vi "take_snapshots.vi"() -> ()   [LabVIEW 2019]
uses:
  <vilib>/userDefined/High Color/IMAQdx.ctl
  <vilib>/vision/driver/IMAQdx.llb/IMAQdx Attribute Type.ctl
  <vilib>/vision/Management.llb/Cast Image 2 Method.ctl
  <vilib>/DAQmx/write.llb/DAQmx Write (Analog DBL 1Chan 1Samp).vi
  <vilib>/DAQmx/read.llb/DAQmx Read (Analog DBL 1Chan 1Samp).vi
  <vilib>/Analysis/baseanly.llb/Mean (DBL).vi
  <vilib>/DAQmx/create/channels.llb/DAQmx Create Channel (AO-Voltage-Basic).vi
  <vilib>/DAQmx/miscellaneous.llb/DAQmx Fill In Error Info.vi
  <vilib>/DAQmx/create/channels.llb/DAQmx Create Channel (AI-Temperature-Thermocouple).vi
  <vilib>/vision/driver/NI_Vision_Acquisition_Software.lvlib
  <resource>/objmgr/imaqdx.rc
  <vilib>/vision/NI_Vision_Development_Module.lvlib
  <vilib>/Analysis/NI_AALBase.lvlib
panel:
  in  "file path (PID voltage)":path
  in  "PID Control 2":bool
  in  "Desired \nTemperature":dbl=20.0 format="%#_13g"
  in  "DC power supply":refnum<visa-resource-name>="COM3"
  out "voltage monitoring constant":dbl format="%#.2g"
  in  "exit PID loop":bool
  in  "Experiment duration\n(min)":dbl
  in  "Snapshot Period\n (min per snapshot)":dbl
  out "Video":bool
  in  "Action":i32(listbox)=1
  out "meanIntensity":dbl[](array[numeric])
  out "varLaplacian":dbl[](array[numeric])
  out "mean":dbl
  out "variance":dbl
  out "Avg Intensity":dbl(graph)=4.716017316017316
  in  "Activate":bool
  out "Var of Laplacian":dbl(graph)=63.940469067936796
  in  "ROI":T1={"Global Rectangle"=[], "Contours"=[{"Contour Type"=0, "ROI Type"=3, "Points"=[231, 86, 235, 90]}, {"Contour Type"=0, "ROI Type"=3, "Points"=[193, 50, 270, 125]}]}
  in  "error in":errorcluster
  in  "File path for video":string="C:\\Users\\Aniket\\Desktop\\mCherry_calibration\\new_lens\\laser_calibration\\laser_and_heating\\"
  in  "Laser profile file path":path=path "C:/Users/Aniket/Desktop/mCherry_calibration/new_lens/laser_calibration/laser_profiles/new_profile.txt"
  in  "Trigger Laser":bool
  in  "Image file path \n(Do not add specify file extension - set to png)":path=path "C:/Users/Aniket/Desktop/mCherry_calibration/new_lens/laser_calibration/laser_profiles.txt"
  out "Current \nTemperature":dbl format="%0.2f"
  out "?":dbl[](graph)=[37.63236695538445]
  out "error out 7":errorcluster
  out "error out 6":errorcluster
  out "error out 5":errorcluster
  out "Exposure Time":dbl
  in  "ON/OFF":bool
  out "error out 3":errorcluster
  in  "LED":dbl(slide) scale=0.0..10.0
  in  "Refresh":bool
  out "Record":bool
  out "Processed Frames per Second":dbl
  out "Acquired Frame Rate":dbl
  out "error out":errorcluster
  out "Camera Display":T2(plugin-control) caption="Image Out"
  in  "Frame Rate":dbl=20.0
  out "Attribute Information Array":T4(array[cluster])
  in  "Session In":T5="cam0"
  # "Camera frame"
  # "Observer frame"
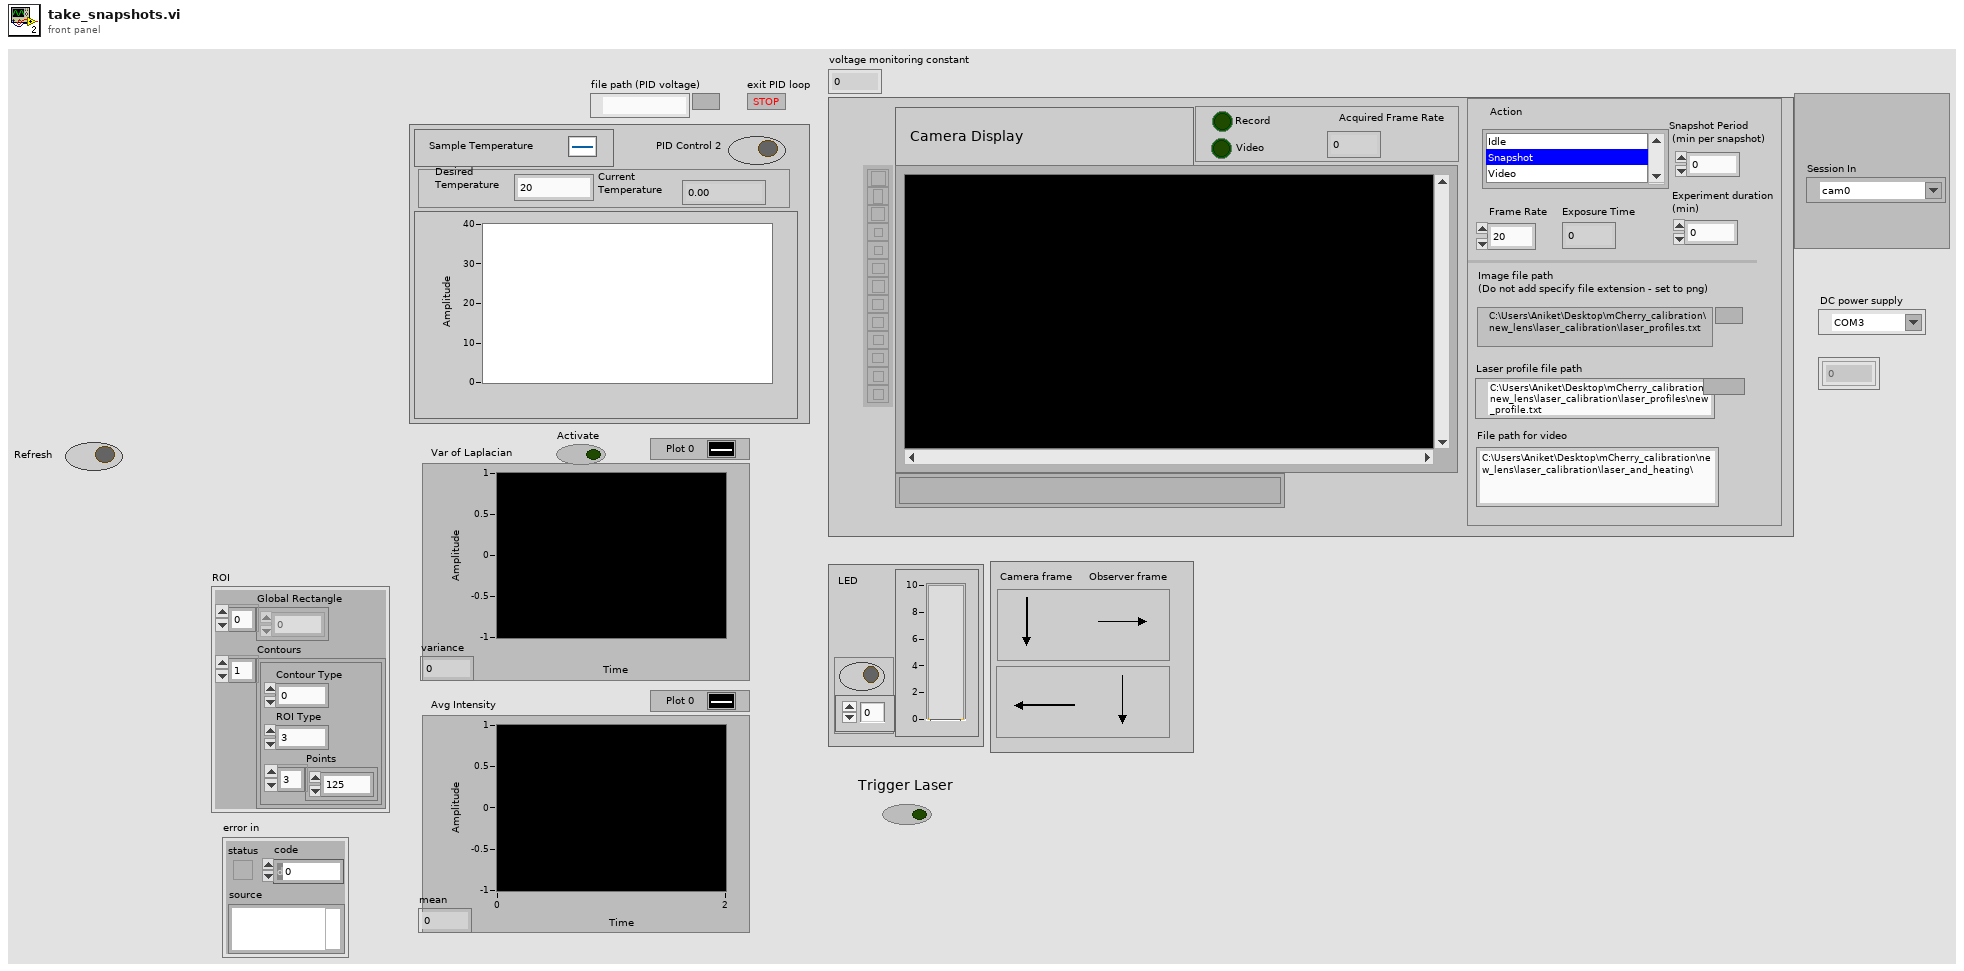
[diagram p1: front panel]
types:
  T1 = cluster{"Global Rectangle":i32[], "Contours":cluster{"Contour Type":u32, "ROI Type":u32, "Points":i32[]}[]}
  T2 = typedef "IMAQ Image.ctl" = refnum<image>
  T3 = typedef "NI_Vision_Acquisition_Software.lvlib/IMAQdx Attribute Type.ctl" = enum32{"U32", "I64", "DBL", "String", "Enum", "Bool", "Command"}
  T4 = cluster{"Attribute Type":T3, "Readable":bool, "Writable":bool, "Attribute Name":string}[]
  T5 = typedef "IMAQdx.ctl" = refnum<k21>
  T6 = enum16{"open", "replace", "create", "open or create", "replace or create", "replace or create with confirmation"}
  T7 = typedef "Image Type" = u32
  T8 = typedef "ROI Descriptor" = cluster{"Global Rectangle":i32[], "Contours":cluster{"ID":enum32{"External", "Internal"}, "Type":u32, "Coordinates":i32[]}[]}
  T9 = typedef "IMAQ Rectangle" = cluster{"Left":i32, "Top":i32, "Right":i32, "Bottom":i32, "Rotation":dbl}
  T10 = typedef "Cast Image 2 Method.ctl" = u32
  T11 = typedef "IMAQ AVI2 Refnum.ctl" = refnum<k20>
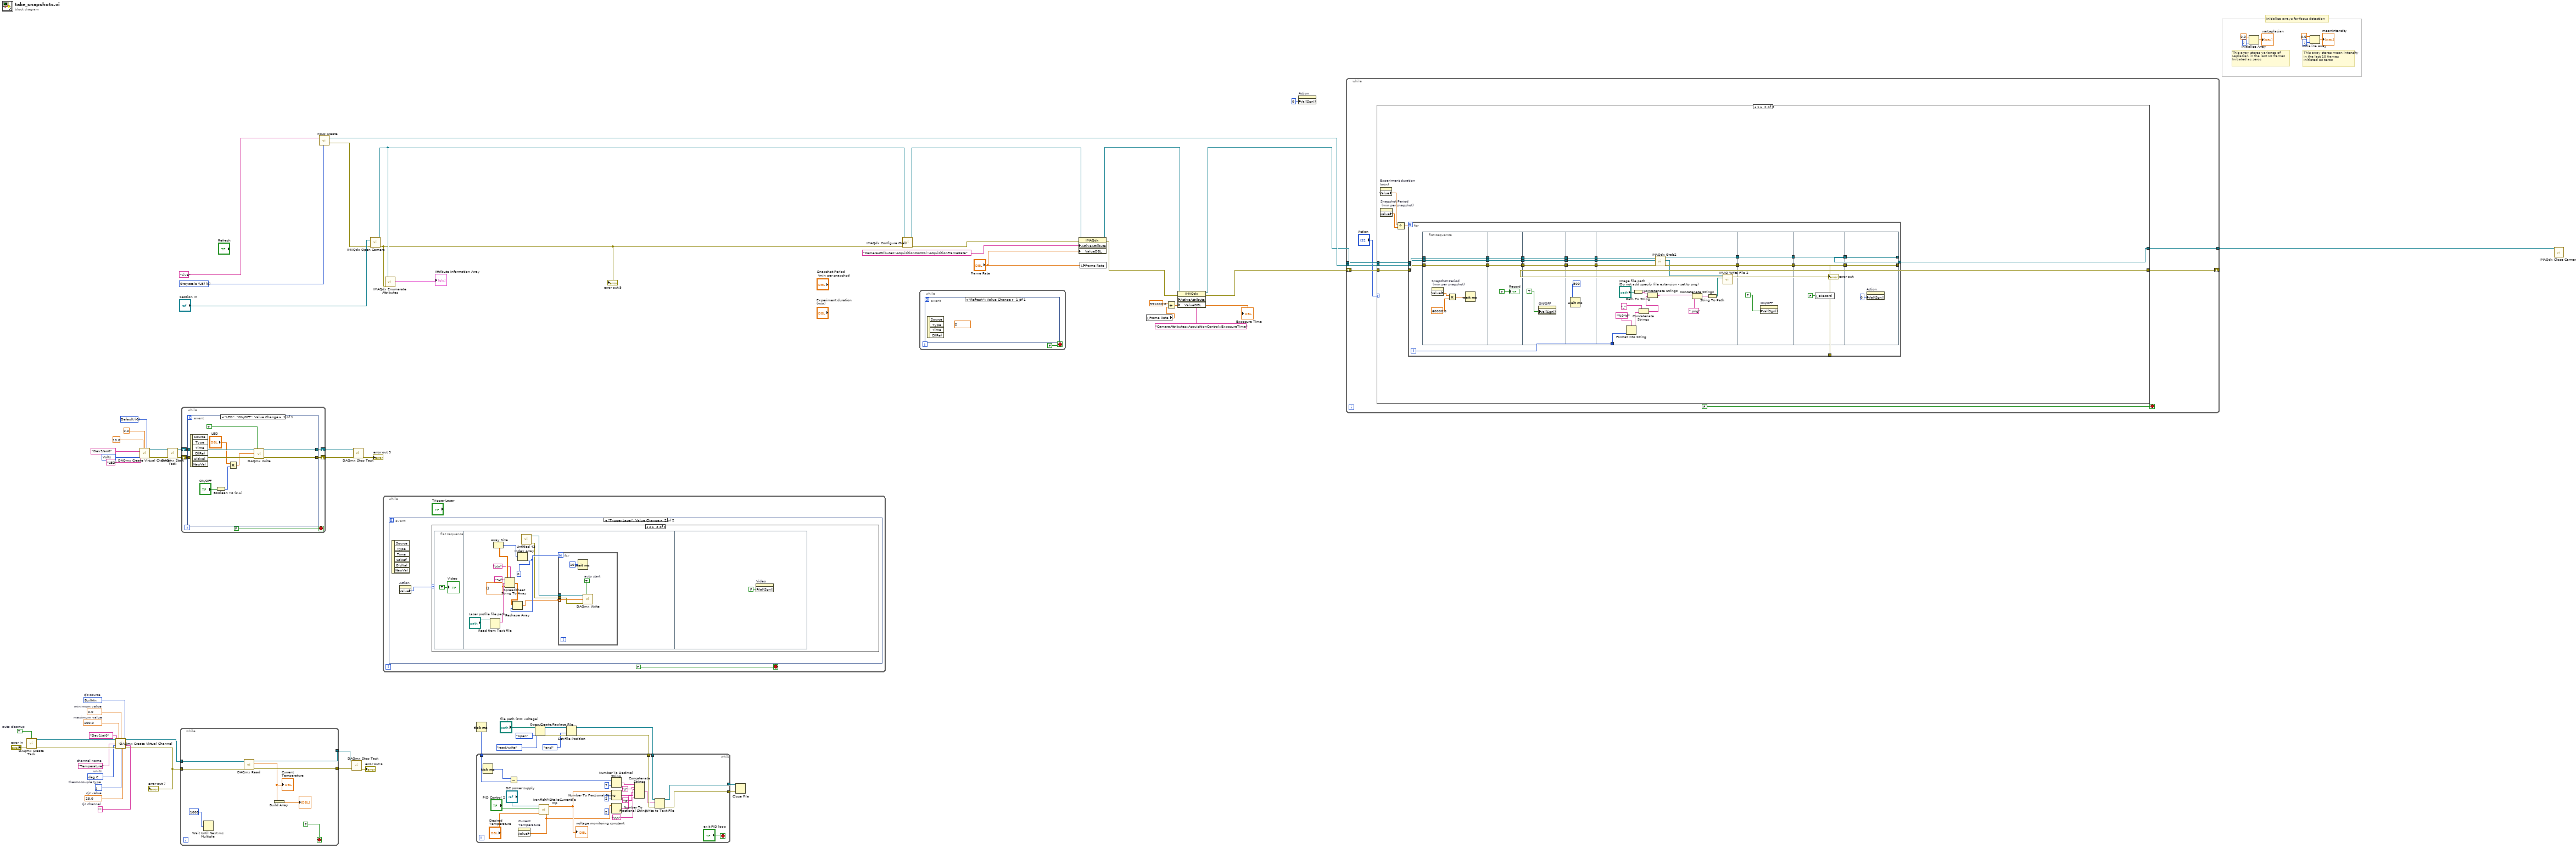
[diagram p0: block diagram]
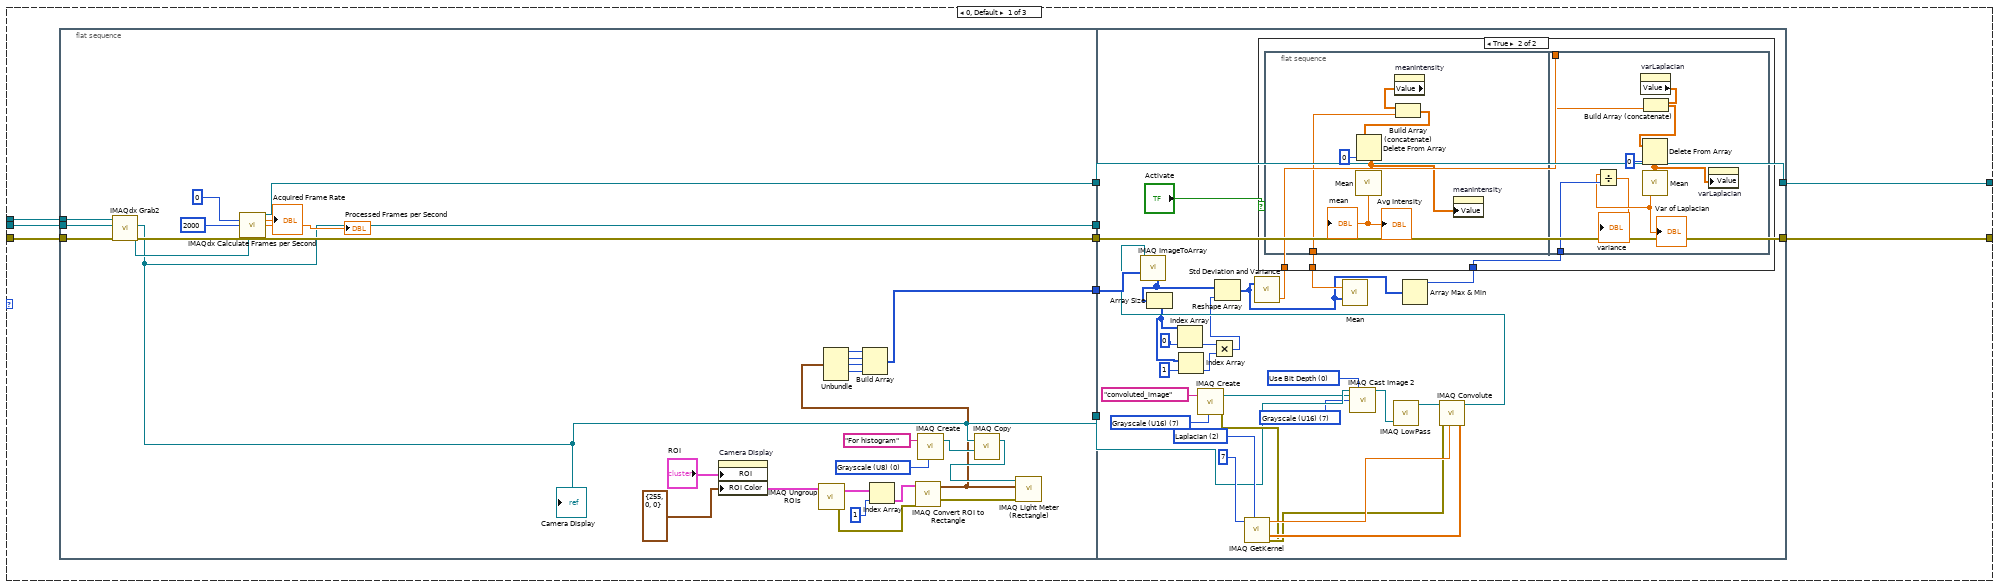
[diagram p2: hidden frame]
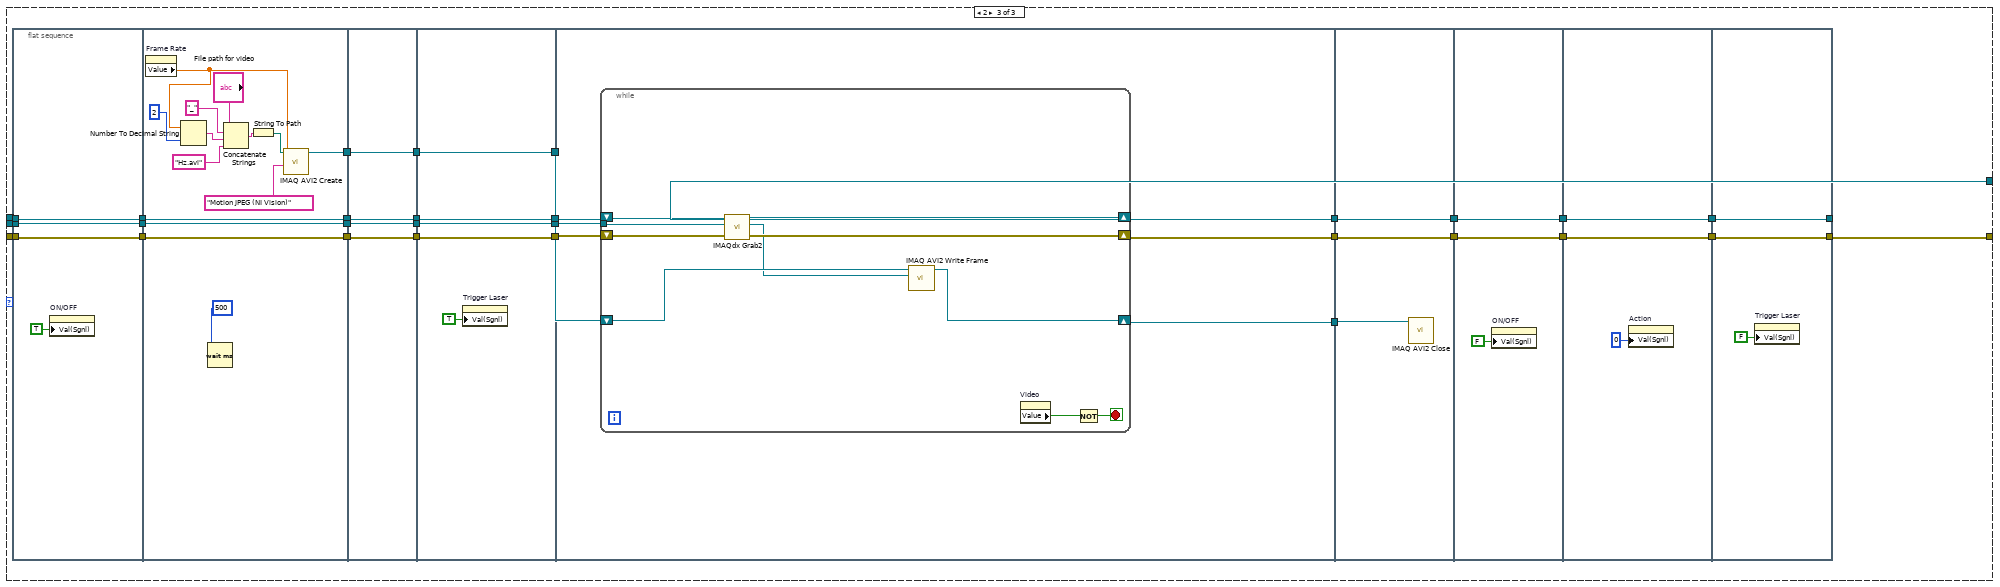
[diagram p4: hidden frame]
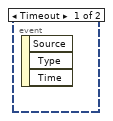
[diagram p5: hidden frame]
diagram:
  w24 = 10200 items=["Built-In"=10200, "Constant Value"=10116, "Channel"=10113]  # cjc source
  w26 = ""  # cjc channel
  w27 = 25.0  # cjc value
  w28 = 10072 items=["J"=10072, "K"=10073, "N"=10077, "R"=10082, "S"=10085, "T"=10086, "B"=10047, "E"=10055]  # thermocouple type
  w29 = 10143 items=["deg C"=10143, "deg F"=10144, "Kelvins"=10325, "deg R"=10145, "From Custom Scale"=10065]  # units
  w25 = "Temperature"  # channel name
  w30 = 0.0  # minimum value
  w31 = 100.0  # maximum value
  w33 = TRUE  # auto cleanup
  w56 = 10348 items=["Volts"=10348, "From Custom Scale"=10065] ("units")
  w58 = -1 items=["Default"=-1, "RSE"=10083, "NRSE"=10078, "Differential"=10106, "Pseudodifferential"=12529] ("input terminal configuration")
  w69 = T7 0 items=["Grayscale (U8)", "Grayscale (I16)", "Grayscale (SGL)", "Complex (CSG)", "RGB (U32)", "HSL (U32)", "RGB (U64)", "Grayscale (U16)"] ("Image Type")
  # "Initialize arrays for focus detection"
  # "This array stores mean intensity in the last 10 frames\nInitiated as zeros"
  # "This array stores variance of Laplacian in the last 10 frames\nInitiated as zeros"
  n1 = call <vilib>:"DAQmx Create Task.vi"("auto cleanup"=w33, "error in"="error in") -> ("task out"=w32:refnum<k21>, "error out"=w34:errorcluster)  [unwired: 12 in]
  n2 = call-poly <vilib>:"DAQmx Create Virtual Channel.vi"("task in"=w32, "maximum value"=w31, "minimum value"=w30, "physical channels"=tag "Dev1/ai0", "cjc source"=w24, "name to assign"=w25, "units"=w29, "cjc channel"=w26, "error in"=w34, "thermocouple type"=w28, "cjc value"=w27) -> ("task out"=w23:refnum<k21>, "error out"=w22:errorcluster)  [unwired: 3 in]
  "error out 7" <- w22
  n3 = call-poly <vilib>:"DAQmx Create Virtual Channel.vi"("maximum value"=10.0, "minimum value"=0.0, "output terminal configuration"=w58, "physical channels"=tag "Dev3/ao0", "name to assign"="LED", "units"=w56) -> ("task out"=w54:refnum<k21>, "error out"=w53:errorcluster)  [unwired: 8 in]
  n4 = call <vilib>:"DAQmx Start Task.vi"("task/channels in"=w54, "error in"=w53) -> ("task out"=w52:refnum<k21>, "error out"=w51:errorcluster)  [unwired: 12 in]
  n5 = while {
    tunnel: w23 -> [w78]
    tunnel: w22 -> [w77]
    tunnel: [w76] -> w38
    tunnel: [w75] -> w37
    stop <- FALSE ("Monitor Temperature") stop-if-true
    n6 = Wait Until Next ms Multiple(millisecond multiple=u32 1000 ("millisecond timer value")) -> ()  [unwired: 1 out]
    n7 = call-poly <vilib>:"DAQmx Read.vi"("task/channels in"=w78, "error in"=w77) -> ("task out"=w76:refnum<k21>, "data"=w72:dbl, "error out"=w75:errorcluster)  [unwired: 11 in]
    "Current \nTemperature" <- w72
    n8 = Build Array(w72) -> (→"?":dbl[])
  }
  n9 = while {
    shift-right: [w82] -> w50
    shift-left: w52 -> [w84]
    shift-right: [w81] -> w49
    shift-left: w51 -> [w83]
    stop <- FALSE stop-if-true
    n10 = event shown="[0] \"LED\", \"ON/OFF\": Value Change" {
      selector: _ -> [_]
      dyn-events: _ -> [_]
      timeout: _ -> [_]
      tunnel: w84 -> [w93]
      tunnel: w83 -> [w92]
      tunnel: [w91] -> w82
      tunnel: [w90] -> w81
      event "LED", "ON/OFF": Value Change {
        n11 = event-data() -> ()  [unwired: 1 in, 6 out]
        n12 = Boolean To (0,1)(Boolean="ON/OFF") -> (0, 1=w86:i16)
        n13 = Multiply(x="LED", y=w86) -> (x*y=w85:dbl)
        n14 = call-poly <vilib>:"DAQmx Write.vi"("task/channels in"=w93, "auto start"=TRUE, "data"=w85, "error in"=w92) -> ("task out"=w91:refnum<k21>, "error out"=w90:errorcluster)  [unwired: 9 in, 1 out]
      }
    }
  }
  n15 = call "IMAQ Create"("Image Name"="Live", "Image Type"=w69) -> ("New Image"=w63:T2, "error out"=w62:errorcluster)  [unwired: 3 in]
  n16 = call <vilib>:"DAQmx Stop Task.vi"("task/channels in"=w38, "error in"=w37) -> ("error out"=→"error out 6":errorcluster)  [unwired: 12 in, 1 out]
  n17 = call <vilib>:"DAQmx Stop Task.vi"("task/channels in"=w50, "error in"=w49) -> ("error out"=→"error out 3":errorcluster)  [unwired: 12 in, 1 out]
  n18 = call <vilib>:"IMAQdx Open Camera.vi"("error in"=w62, "Session In"="Session In") -> ("error out"=w67:errorcluster, "Session Out"=w68:T5)  [unwired: 8 in]
  "error out 5" <- w67
  n19 = while {
    stop <- FALSE stop-if-true
    n20 = event shown="[1] \"Trigger Laser\": Value Change" {
      selector: _ -> [_ _]
      dyn-events: _ -> [_ _]
      timeout: _ -> [_ _]
      event Timeout {
        n21 = event-data() -> ()  [unwired: 1 in, 3 out]
      }
      event "Trigger Laser": Value Change {
        n22 = event-data() -> ()  [unwired: 1 in, 6 out]
        n23 = property on="Action" class="LstBox (strict)"() -> ("Value"=w95:i32)  [unwired: 2 in, 2 out]
        n24 = case shown="2" w95 {
          frame 0, Default {
          }
          frame 1 {
          }
          frame 2 {
            n25 = flat-sequence {
              frame #0 {
                "Video" <- TRUE ("Video")
              }
              frame #1 {
                n26 = Read from Text File(file (use dialog)="Laser profile file path") -> (text=w104:string)  [unwired: 3 in, 3 out]
                n27 = Spreadsheet String To Array(delimiter (Tab)="\r\n", format string="%f", spreadsheet string=w104, array type (2D Dbl)=dbl[][] []) -> (array=w106:dbl[][])
                n28 = Array Size(array=w106) -> (size(s)=w105:i32[])
                n29 = Index Array(array=w105, index=0) -> (element=w108:i32)
                n30 = Reshape Array(w106, w108) -> (w107:dbl[])
                n31 = call "Untitled 43.vi"() -> ("error out"=w97:errorcluster, "task out"=w98:refnum<k21>)  [unwired: 10 in]
                n32 = for {
                  N: w108 -> [_]
                  tunnel: w107 -> [w109] mode=indexing
                  tunnel: w98 -> [w111]
                  tunnel: w97 -> [w110]
                  w112 = TRUE  # auto start
                  n33 = Wait (ms)(milliseconds to wait=u32 10) -> ()  [unwired: 1 out]
                  n34 = call-poly <vilib>:"DAQmx Write.vi"("task/channels in"=w111, "auto start"=w112, "data"=w109, "error in"=w110) -> ()  [unwired: 9 in, 3 out]
                }
              }
              frame #2 {
                n35 = property on="Video" class="Bool (strict)"("Val(Sgnl)"=FALSE ("Value (Signaling)")) -> ()  [unwired: 2 in, 2 out]
              }
            }
          }
        }
      }
    }
  }
  n36 = call <vilib>:"IMAQdx Enumerate Attributes.vi"("error in"=w67, "Session In"=w68) -> ("Attribute Information Array"=→"Attribute Information Array":T4)  [unwired: 7 in, 2 out]
  n37 = Tick Count (ms)() -> (millisecond timer value=w11:u32)
  n38 = Open/Create/Replace File(file path (use dialog)="file path (PID voltage)", operation (0:open)=T6."open", access (0:read/write)=enum16{"read/write", "read-only", "write-only"}."read/write") -> (refnum out=w7:refnum<file>, error out=w8:errorcluster)  [unwired: 3 in, 1 out]
  n39 = Set File Position(refnum=w7, from (0:start)=enum16{"start", "end", "current"}."end", error in=w8) -> (refnum out=w5:refnum<file>, error out=w4:errorcluster)  [unwired: 1 in]
  n40 = while {
    tunnel: w11 -> [w133]
    tunnel: w5 -> [w117]
    tunnel: w4 -> [w116]
    tunnel: [w118] -> w3
    tunnel: [w119] -> w2
    stop <- "exit PID loop" stop-if-true
    n41 = Tick Count (ms)() -> (millisecond timer value=w134:u32)
    n42 = Subtract(x=w134, y=w133) -> (x-y=w131:u32)
    n43 = property on="Current \nTemperature" class="DigNum (strict)"() -> ("Value"=w123:dbl)  [unwired: 2 in, 2 out]
    n44 = call "IronFishPIDtakeCurrentTemp.vi"(0:"DC power supply", "Switch"="PID Control 2", "Desired Temp"="Desired \nTemperature", "Current Temp"=w123) -> ("voltage monitoring constant"=w132:dbl)  [unwired: 4 in]
    "voltage monitoring constant" <- w132
    n45 = Number To Decimal String(number=w131, width (-)=i16 7) -> (decimal integer string=w129:string)
    n46 = Number To Fractional String(number=w132, precision (6)=i16 2) -> (F-format string=w127:string)  [unwired: 2 in]
    n47 = Number To Fractional String(number=w123, precision (6)=i16 2) -> (F-format string=w121:string)  [unwired: 2 in]
    n48 = Concatenate Strings(w129, "\t", w127, "\t", w121, "\r\n") -> (w115:string)
    n49 = Write to Text File(file (use dialog)=w117, text=w115, error in=w116) -> (refnum out=w118:refnum<file>, error out=w119:errorcluster)  [unwired: 1 in, 1 out]
  }
  n50 = Close File(refnum=w3, error in=w2) -> ()  [unwired: 2 out]
  n51 = call <vilib>:"IMAQdx Configure Grab.vi"("error in"=w67, "Session In"=w68) -> ("error out"=w65:errorcluster, "Session Out"=w47:T5)  [unwired: 8 in]
  n52 = while {
    stop <- FALSE stop-if-true
    n53 = event shown="[0] \"Refresh\": Value Change" {
      selector: _ -> [_]
      dyn-events: _ -> [_]
      timeout: _ -> [_]
      event "Refresh": Value Change {
        (unwired) dbl[] [] ("History Data")
        n54 = event-data() -> ()  [unwired: 1 in, 4 out]
      }
    }
  }
  n55 = property class="IMAQdx"(reference=w47, error in=w65, "ActiveAttribute"="CameraAttributes::AcquisitionControl::AcquisitionFrameRate", "ValueDBL"="Frame Rate") -> (reference out=w42:T5, error out=w40:errorcluster)
  n56 = local write "Frame Rate"("Frame Rate") -> ()
  n57 = local read "Frame Rate"() -> (w44:dbl)
  n58 = Divide(x=991000.0, y=w44) -> (x/y=w43:dbl)
  "Exposure Time" <- w43
  n59 = property class="IMAQdx"(reference=w42, error in=w40, "ActiveAttribute"="CameraAttributes::AcquisitionControl::ExposureTime", "ValueDBL"=w43) -> (reference out=w41:T5, error out=w39:errorcluster)
  n60 = property on="Action" class="LstBox (strict)"("Val(Sgnl)"=0 ("Value (Signaling)")) -> ()  [unwired: 2 in, 2 out]
  n61 = while {
    tunnel: w41 -> [w145]
    tunnel: w63 -> [w143]
    shift-right: [w142] -> w12
    shift-left: w39 -> [w144]
    tunnel: [w139] -> w14
    stop <- FALSE ("Stop") stop-if-true
    n62 = case shown="1" "Action" {
      tunnel: w145 -> [w155 w238 w335]
      tunnel: w144 -> [w154 w236 w333]
      tunnel: w143 -> [w153 w237 w334]
      tunnel: [w152 w235 w331] -> w142
      tunnel: [w151 w234 w332] -> w139
      frame 0, Default {
        n63 = flat-sequence {
          tunnel: w155 -> [w183]
          tunnel: w154 -> [w182]
          tunnel: w153 -> [w181]
          tunnel: [w180] -> w150
          tunnel: [w178] -> w149
          tunnel: [w165] -> w148
          tunnel: [w165] -> w147
          tunnel: [w157] -> w146
          tunnel: [w212] -> w151
          tunnel: [w213] -> w152
          tunnel: w150 -> [w213]
          tunnel: w149 -> [w212]
          tunnel: w148 -> [_]
          tunnel: w147 -> [w193]
          tunnel: w146 -> [w203]
          frame #0 {
            w166 = T7 0 items=["Grayscale (U8)", "Grayscale (I16)", "Grayscale (SGL)", "Complex (CSG)", "RGB (U32)", "HSL (U32)", "RGB (U64)", "Grayscale (U16)"] ("Image Type")
            n64 = call <vilib>:"IMAQdx Grab2.vi"("error in"=w182, "Image In"=w181, "Session In"=w183) -> ("error out"=w180:errorcluster, "Image Out"=w165:T2, "Session Out"=w179:T5)  [unwired: 5 in, 1 out]
            "Camera Display" <- w165
            n65 = call <vilib>:"IMAQdx Calculate Frames per Second.vi"("Session In"=w179, "Buffer Number"=u32 0, "Minimum Display Update Interval (ms)"=u32 2000) -> ("Session Out"=w178:T5, "Acquired Frames per Second"=→"Acquired Frame Rate":dbl, "Processed Frames per Second"=→"Processed Frames per Second":dbl)  [unwired: 6 in, 4 out]
            n66 = property on="Camera Display" class="ImageControl"("ROI"="ROI", "ROI Color"=cluster{"Red":u8, "Green":u8, "Blue":u8} {"Red"=255, "Green"=0, "Blue"=0}) -> ()  [unwired: 2 in, 2 out]
            n67 = call "IMAQ Ungroup ROIs"("ROI Descriptor"="ROI") -> ("error out"=w169:errorcluster, "ROI Descriptors out"=w172:T8[])  [unwired: 3 in]
            n68 = Index Array(array=w172, index=1) -> (element=w170:T8)
            n69 = call "IMAQ Convert ROI to Rectangle"("error in (no error)"=w169, "ROI Descriptor"=w170) -> ("error out"=w168:errorcluster, "Rectangle"=w162:T9)  [unwired: 7 in]
            n70 = Unbundle(w162) -> ("Left"=w161:i32, "Top"=w160:i32, "Right"=w159:i32, "Bottom"=w158:i32)  [unwired: 1 out]
            n71 = Build Array(w161, w160, w159, w158) -> (w157:i32[])
            n72 = call "IMAQ Create"("Image Name"="For histogram", "Image Type"=w166) -> ("New Image"=w164:T2)  [unwired: 3 in, 1 out]
            n73 = call "IMAQ Copy"("Image Dst"=w164, "Image Src"=w165) -> ("Image Dst Out"=w163:T2)  [unwired: 4 in, 1 out]
            n74 = call "IMAQ Light Meter (Rectangle)"("error in (no error)"=w168, "Rectangle"=w162, "Image"=w163) -> ()  [unwired: 4 in, 5 out]
          }
          frame #1 {
            w189 = T7 7 items=["Grayscale (U8)", "Grayscale (I16)", "Grayscale (SGL)", "Complex (CSG)", "RGB (U32)", "HSL (U32)", "RGB (U64)", "Grayscale (U16)"] ("Image Type")
            w192 = T10 0 items=["Use Bit Depth", "Shift", "Use Lookup Table"] ("Method")
            w208 = u16 2 items=["Gradient"=1, "Laplacian"=2, "Smoothing"=3, "Gaussian"=4] ("Kernel Family")
            w210 = T7 7 items=["Grayscale (U8)", "Grayscale (I16)", "Grayscale (SGL)", "Complex (CSG)", "RGB (U32)", "HSL (U32)", "RGB (U64)", "Grayscale (U16)"] ("Image Type")
            n75 = call "IMAQ Create"("Image Name"="convoluted_image", "Image Type"=w210) -> ("New Image"=w191:T2, "error out"=w204:errorcluster)  [unwired: 3 in]
            n76 = call "IMAQ GetKernel"("Kernel Family"=w208, "error in (no error)"=w204, "Kernel Size (3,5,...)"=7) -> ("error out"=w205:errorcluster, "Kernel"=w206:sgl[][], "Divider"=w207:sgl)  [unwired: 5 in, 1 out]
            n77 = call "IMAQ Cast Image 2"("Image Src"=w193, "Method"=w192, "Image Dst"=w191, "Image Type"=w189) -> ("Image Dst Out"=w190:T2)  [unwired: 10 in, 1 out]
            n78 = call "IMAQ LowPass"("Image Src"=w190) -> ("Image Dst Out"=w194:T2)  [unwired: 6 in, 1 out]
            n79 = call "IMAQ Convolute"("Kernel"=w206, "Divider (kernel sum)"=w207, "error in (no error)"=w205, "Image Src"=w194) -> ("Image Dst Out"=w202:T2)  [unwired: 6 in, 1 out]
            n80 = call "IMAQ ImageToArray"("Optional Rectangle"=w203, "Image"=w202) -> ("Image Pixels (U16)"=w187:u16[][])  [unwired: 2 in, 4 out]
            n81 = Array Size(array=w187) -> (size(s)=w188:i32[])
            n82 = Index Array(array=w188, index=0 ("index (row)")) -> (element=w199:i32)
            n83 = Index Array(array=w188, index=1) -> (element=w198:i32)
            n84 = Multiply(x=w199, y=w198) -> (x*y=w186:i32)
            n85 = Reshape Array(w187, w186) -> (w185:u16[])
            n86 = call <vilib>:"Std Deviation and Variance.vi"("X"=w185) -> ("variance"=w196:dbl)  [unwired: 1 in, 2 out]
            n87 = call-poly <vilib>:"Mean.vi"("X"=w185) -> ("mean"=w195:dbl)  [unwired: 1 out]
            n88 = Array Max & Min(array=w185) -> (max value=w184:u16)  [unwired: 3 out]
            n89 = case shown="True" "Activate" {
              tunnel: w196 -> [_ w215]
              tunnel: w195 -> [_ w216]
              tunnel: w184 -> [_ w214]
              frame False {
              }
              frame True {
                n90 = flat-sequence {
                  tunnel: w216 -> [w219]
                  tunnel: w215 -> [w225]
                  tunnel: w214 -> [w230]
                  frame #0 {
                    n91 = property on="meanIntensity" class="Arr (strict)"() -> ("Value"=w220:dbl[])  [unwired: 2 in, 2 out]
                    n92 = Build Array (concatenate)(w220, w219) -> (w218:dbl[])
                    n93 = Delete From Array(array=w218, index=0) -> (array with subset deleted=w217:dbl[])  [unwired: 1 in, 1 out]
                    n94 = call-poly <vilib>:"Mean.vi"("X"=w217) -> ("mean"=→"Avg Intensity" →"mean":dbl)  [unwired: 1 out]
                    n95 = property on="meanIntensity" class="Arr (strict)"("Value"=w217) -> ()  [unwired: 2 in, 2 out]
                  }
                  frame #1 {
                    n96 = property on="varLaplacian" class="Arr (strict)"() -> ("Value"=w226:dbl[])  [unwired: 2 in, 2 out]
                    n97 = Build Array (concatenate)(w226, w225) -> (w224:dbl[])
                    n98 = Delete From Array(array=w224, index=0) -> (array with subset deleted=w223:dbl[])  [unwired: 1 in, 1 out]
                    n99 = call-poly <vilib>:"Mean.vi"("X"=w223) -> ("mean"=w229:dbl)  [unwired: 1 out]
                    "Var of Laplacian" <- w229
                    n100 = Divide(x=w229, y=w230) -> (x/y=→"variance":dbl)
                    n101 = property on="varLaplacian" class="Arr (strict)"("Value"=w223) -> ()  [unwired: 2 in, 2 out]
                  }
                }
              }
            }
          }
        }
      }
      frame 1 {
        n102 = property on="Experiment duration\n(min)" class="DigNum (strict)"() -> ("Value"=w232:dbl)  [unwired: 2 in, 2 out]
        n103 = property on="Snapshot Period\n (min per snapshot)" class="DigNum (strict)"() -> ("Value"=w231:dbl)  [unwired: 2 in, 2 out]
        n104 = Divide(x=w232, y=w231) -> (x/y=w233:dbl)
        n105 = for {
          N: w233 -> [_]
          tunnel: w238 -> [w247]
          tunnel: w237 -> [w246]
          tunnel: w236 -> [w245]
          tunnel: [w244] -> w235
          tunnel: [w243] -> w234
          i -> [w242]
          n106 = flat-sequence {
            tunnel: w247 -> [w266]
            tunnel: w246 -> [w267]
            tunnel: w245 -> [w268]
            tunnel: [w268] -> w241
            tunnel: [w267] -> w240
            tunnel: [w266] -> w239
            tunnel: [w272] -> w262
            tunnel: [w271] -> w261
            tunnel: [w270] -> w260
            tunnel: w239 -> [w270]
            tunnel: w240 -> [w271]
            tunnel: w241 -> [w272]
            tunnel: [w276] -> w259
            tunnel: [w275] -> w258
            tunnel: [w274] -> w257
            tunnel: w262 -> [w276]
            tunnel: w261 -> [w275]
            tunnel: w260 -> [w274]
            tunnel: w259 -> [w280]
            tunnel: [w280] -> w256
            tunnel: w258 -> [w279]
            tunnel: [w279] -> w255
            tunnel: w257 -> [w278]
            tunnel: [w278] -> w254
            tunnel: [w293] -> w253
            tunnel: [w297] -> w252
            tunnel: w256 -> [w296]
            tunnel: w255 -> [w295]
            tunnel: w254 -> [w294]
            tunnel: w242 -> [w281]
            tunnel: w253 -> [w300]
            tunnel: [w300] -> w251
            tunnel: w252 -> [w299]
            tunnel: [w299] -> w250
            tunnel: w251 -> [w303]
            tunnel: w250 -> [w302]
            tunnel: [w303] -> w249
            tunnel: [w302] -> w248
            tunnel: [w306] -> w244
            tunnel: [w304] -> w243
            tunnel: w249 -> [w304]
            tunnel: w248 -> [w306]
            frame #0 {
              n107 = property on="Snapshot Period\n (min per snapshot)" class="DigNum (strict)"() -> ("Value"=w265:dbl)  [unwired: 2 in, 2 out]
              n108 = Multiply(x=w265, y=60000.0) -> (x*y=w263:dbl)
              n109 = Wait (ms)(milliseconds to wait=w263) -> ()  [unwired: 1 out]
            }
            frame #1 {
              "Record" <- TRUE ("Record")
            }
            frame #2 {
              n110 = property on="ON/OFF" class="Bool (strict)"("Val(Sgnl)"=TRUE ("ON/OFF")) -> ()  [unwired: 2 in, 2 out]
            }
            frame #3 {
              n111 = Wait (ms)(milliseconds to wait=u32 500) -> ()  [unwired: 1 out]
            }
            frame #4 {
              n112 = Format Into String(format string="%04d", w281) -> (resulting string=w282:string)  [unwired: 2 in, 1 out]
              n113 = Path To String(path="Image file path \n(Do not add specify file extension - set to png)") -> (string=w289:string)
              n114 = Concatenate Strings("_" ("string"), w282) -> (w288:string)
              n115 = Concatenate Strings(w289, w288) -> (w287:string)
              n116 = call <vilib>:"IMAQdx Grab2.vi"("error in"=w296, "Image In"=w295, "Session In"=w294) -> ("error out"=w297:errorcluster, "Image Out"=w292:T2, "Session Out"=w293:T5)  [unwired: 5 in, 1 out]
              n117 = Concatenate Strings(w287, ".png" ("string")) -> (w285:string)
              n118 = String To Path(string=w285) -> (path=w284:path)
              n119 = call-poly "IMAQ Write File 2"("File Path"=w284, "Image"=w292) -> ()  [unwired: 8 in, 2 out]
            }
            frame #5 {
              n120 = property on="ON/OFF" class="Bool (strict)"("Val(Sgnl)"=FALSE ("ON/OFF")) -> ()  [unwired: 2 in, 2 out]
            }
            frame #6 {
              n121 = local write "Record"(FALSE ("Record")) -> ()
            }
            frame #7 {
              n122 = property on="Action" class="LstBox (strict)"("Val(Sgnl)"=0 ("Value (Signaling)")) -> ()  [unwired: 2 in, 2 out]
            }
          }
        }
      }
      frame 2 {
        n123 = flat-sequence {
          tunnel: w333 -> [w337]
          tunnel: w334 -> [w338]
          tunnel: w335 -> [w339]
          tunnel: [w339] -> w330
          tunnel: [w338] -> w329
          tunnel: [w337] -> w328
          tunnel: w330 -> [w353]
          tunnel: [w353] -> w327
          tunnel: w329 -> [w352]
          tunnel: [w352] -> w325
          tunnel: w328 -> [w351]
          tunnel: [w351] -> w323
          tunnel: [w348] -> w316
          tunnel: w327 -> [w357]
          tunnel: [w357] -> w326
          tunnel: w325 -> [w356]
          tunnel: [w356] -> w324
          tunnel: w323 -> [w355]
          tunnel: [w355] -> w322
          tunnel: [w354] -> w317
          tunnel: w316 -> [w354]
          tunnel: w326 -> [w359]
          tunnel: w324 -> [w360]
          tunnel: w322 -> [w361]
          tunnel: [w361] -> w321
          tunnel: [w360] -> w320
          tunnel: [w359] -> w319
          tunnel: [w358] -> w318
          tunnel: w317 -> [w358]
          tunnel: w321 -> [w368]
          tunnel: w320 -> [w367]
          tunnel: w319 -> [w366]
          tunnel: [w364] -> w315
          tunnel: [w365] -> w314
          tunnel: [w369] -> w313
          tunnel: w318 -> [w363]
          tunnel: w315 -> [w382]
          tunnel: [w382] -> w310
          tunnel: w314 -> [w381]
          tunnel: [w381] -> w312
          tunnel: w313 -> [w380]
          tunnel: w312 -> [w385]
          tunnel: [w385] -> w311
          tunnel: w310 -> [w384]
          tunnel: [w384] -> w309
          tunnel: w311 -> [w387]
          tunnel: w309 -> [w388]
          tunnel: [w388] -> w308
          tunnel: [w387] -> w307
          tunnel: [w390] -> w331
          tunnel: [w391] -> w332
          tunnel: w308 -> [w391]
          tunnel: w307 -> [w390]
          frame #0 {
            n124 = property on="ON/OFF" class="Bool (strict)"("Val(Sgnl)"=TRUE ("Value (Signaling)")) -> ()  [unwired: 2 in, 2 out]
          }
          frame #1 {
            n125 = property on="Frame Rate" class="DigNum (strict)"() -> ("Value"=w346:dbl)  [unwired: 2 in, 2 out]
            n126 = Number To Decimal String(number=w346, width (-)=i16 2) -> (decimal integer string=w341:string)
            n127 = Wait (ms)(milliseconds to wait=u32 500) -> ()  [unwired: 1 out]
            n128 = Concatenate Strings("File path for video", "_" ("string"), w341, "Hz.avi" ("string")) -> (w343:string)
            n129 = String To Path(string=w343) -> (path=w344:path)
            n130 = call "IMAQ AVI2 Create"("Codec"="Motion JPEG (NI Vision)", "Frames Per Second"=w346, "AVI Path"=w344) -> ("AVI Refnum"=w348:T11)  [unwired: 7 in, 1 out]
          }
          frame #2 {
          }
          frame #3 {
            n131 = property on="Trigger Laser" class="Bool (strict)"("Val(Sgnl)"=TRUE ("Value (Signaling)")) -> ()  [unwired: 2 in, 2 out]
          }
          frame #4 {
            n132 = while {
              tunnel: w367 -> [w377]
              shift-right: [w375] -> w365
              shift-left: w368 -> [w378]
              shift-right: [w374] -> w364
              shift-left: w366 -> [w376]
              shift-right: [w379] -> w369
              shift-left: w363 -> [w373]
              stop <- w371 stop-if-true
              n133 = call <vilib>:"IMAQdx Grab2.vi"("error in"=w378, "Image In"=w377, "Session In"=w376) -> ("error out"=w375:errorcluster, "Image Out"=w372:T2, "Session Out"=w374:T5)  [unwired: 5 in, 1 out]
              n134 = call "IMAQ AVI2 Write Frame"("Image"=w372, "AVI Refnum"=w373) -> ("AVI Refnum (duplicate)"=w379:T11)  [unwired: 7 in, 2 out]
              n135 = property on="Video" class="Bool (strict)"() -> ("Value"=w370:bool)  [unwired: 2 in, 2 out]
              n136 = Not(x=w370) -> (.not. x?=w371:bool)
            }
          }
          frame #5 {
            n137 = call "IMAQ AVI2 Close"("AVI Refnum"=w380) -> ()  [unwired: 10 in, 1 out]
          }
          frame #6 {
            n138 = property on="ON/OFF" class="Bool (strict)"("Val(Sgnl)"=FALSE ("Value (Signaling)")) -> ()  [unwired: 2 in, 2 out]
          }
          frame #7 {
            n139 = property on="Action" class="LstBox (strict)"("Val(Sgnl)"=0 ("Value (Signaling)")) -> ()  [unwired: 2 in, 2 out]
          }
          frame #8 {
            n140 = property on="Trigger Laser" class="Bool (strict)"("Val(Sgnl)"=FALSE ("Value (Signaling)")) -> ()  [unwired: 2 in, 2 out]
          }
        }
      }
    }
  }
  "error out" <- w12
  n141 = Initialize Array(0.0 ("element"), 7 ("dimension size")) -> (→"varLaplacian":dbl[])
  n142 = Initialize Array(0.0 ("element"), 7 ("dimension size")) -> (→"meanIntensity":dbl[])
  n143 = call <vilib>:"IMAQdx Close Camera.vi"("Session In"=w14) -> ()  [unwired: 10 in, 1 out]
